vi "Emilio_tres.vi"() -> ()   [LabVIEW 2024]
panel:
  in  "stop":bool
  in  "Numeric":dbl
  out "Waveform Graph":dbl[](graph)
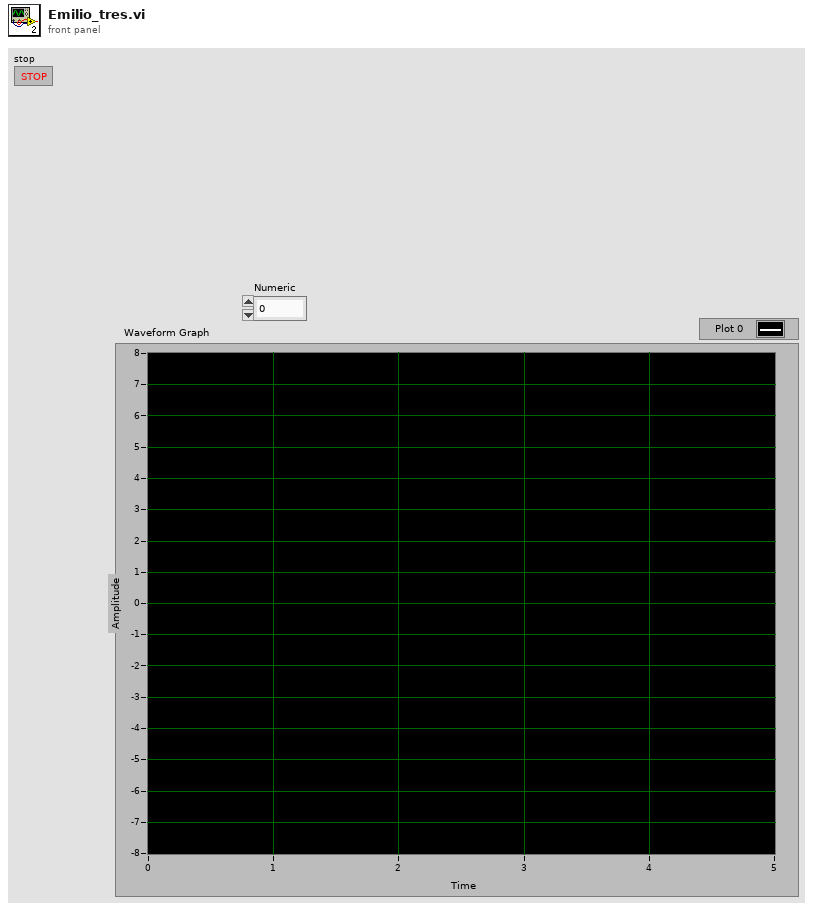
[diagram p1: front panel]
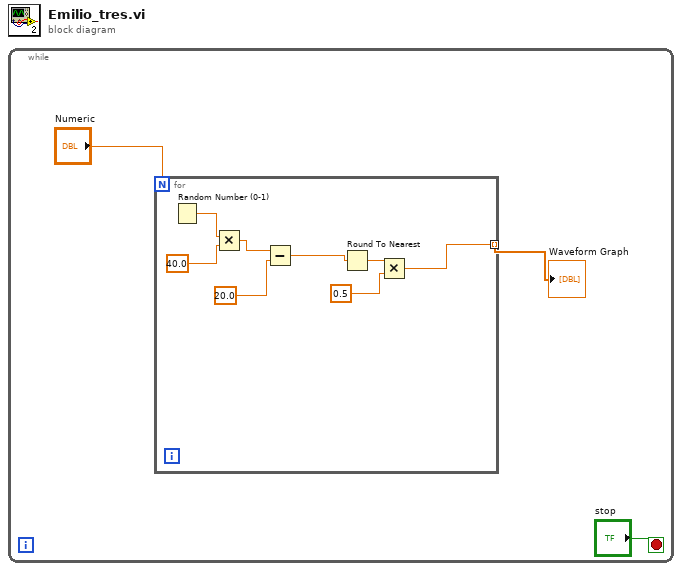
[diagram p0: block diagram]
diagram:
  n1 = while {
    stop <- "stop" stop-if-true
    n2 = for {
      N: "Numeric" -> [_]
      tunnel: [w7] -> w2 mode=indexing
      n3 = Random Number (0-1)() -> (number: 0 to 1=w11:dbl)
      n4 = Multiply(x=w11, y=40.0) -> (x*y=w6:dbl)
      n5 = Subtract(x=w6, y=20.0) -> (x-y=w4:dbl)
      n6 = Round To Nearest(number=w4) -> (nearest integer value=w9:dbl)
      n7 = Multiply(x=w9, y=0.5) -> (x*y=w7:dbl)
    }
    "Waveform Graph" <- w2
  }
